vi "Dynamic call-Coordinates list window.vi"(8 "error in (no error)":errorcluster) -> (0 "error out":errorcluster)   [LabVIEW 2013]
uses:
  Windows/Coordinates list window/Globals/Coord window-Globals.vi
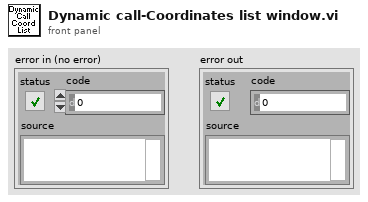
[diagram p1: front panel]
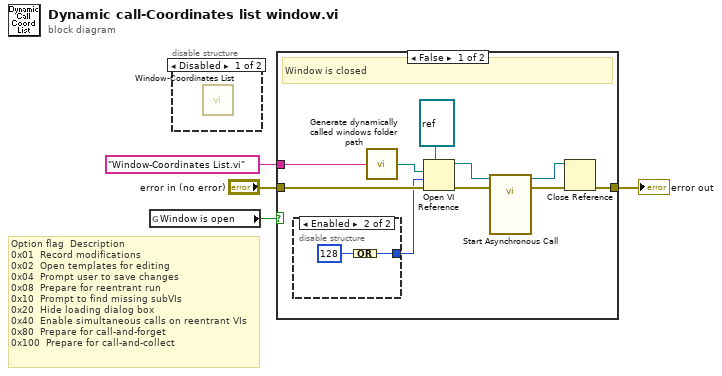
[diagram p0: block diagram]
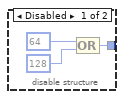
[diagram p2: hidden frame]
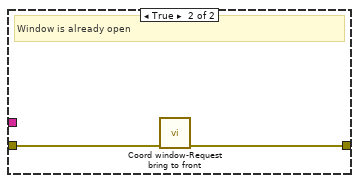
[diagram p3: hidden frame]
diagram:
  # "Option flag \tDescription\n0x01 \tRecord modifications\n0x02 \tOpen templates for editing\n0x04 \tPrompt user to save changes\n0x08 \tPrepare for reentrant run\n0x10 \tPrompt to find missing subVIs\n0x20 \tHide loading dialog box\n0x40 \tEnable simultaneous calls on reentrant VIs\n0x80 \tPrepare for call-and-forget\n0x100 \tPrepare for call-and-collect"
  n1 = global read "Coord window-Globals.vi" "Window is open"() -> (w1:bool)
  n2 = disable-structure shown="Disabled" {
    frame Disabled {
      n3 = call "Window-Coordinates List.vi"() -> ()  [unwired: 12 in]
    }
    frame Enabled {
    }
  }
  n4 = case shown="False" w1 {
    tunnel: "error in (no error)" -> [w14 w21]
    tunnel: [w13 w20] -> w4
    tunnel: "Window-Coordinates List.vi" ("Error Source") -> [w11 _]
    frame False {
      # "Window is closed"
      n5 = disable-structure shown="Enabled" {
        disable-tunnel: [w17 w19] -> w8
        frame Disabled {
          n6 = Compound Arithmetic op=OR(64, 128) -> (w17:i32)
        }
        frame Enabled {
          n7 = Compound Arithmetic op=OR(128) -> (w19:i32)
        }
      }
      n8 = call "Generate dynamically called windows folder path.vi"("name of dynamically called VI"=w11) -> ("Dynamically called VI path"=w12:path)
      n9 = Open VI Reference(type specifier VI Refnum (for type only)=refnum<vi> refnum, vi path=w12, options=w8, error in (no error)=w14) -> (vi reference=w9:refnum<vi>, error out=w10:errorcluster)  [unwired: 2 in]
      n10 = call-by-ref "Start Asynchronous Call"(reference=w9, error in=w10) -> (reference out=w5:refnum<vi>, error out=w6:errorcluster)  [unwired: 12 in]
      n11 = Close Reference(reference=w5, error in (no error)=w6) -> (error out=w13:errorcluster)
    }
    frame True {
      # "Window is already open"
      n12 = call "Coord window-Request bring to front.vi"("error in (no error)"=w21) -> ("error out"=w20:errorcluster)  [unwired: 10 in]
    }
  }
  "error out" <- w4
